vi "Log CAN messages.vi"(8 "error in":errorcluster, 9 "Period":i64, 10 "CAN Session In":T1, 11 "tdms file in":refnum<k34>) -> (0 "error out":errorcluster, 2 "CAN Session Out":T1, 3 "tdms file out":refnum<k34>)   [LabVIEW 2016]
uses:
  Program Files (x86)/National Instruments/LabVIEW 2016/examples/robotics/EPOS2 CANOpen Driver/Low Level VIs/Typedefs/CAN Refnum.ctl
  Program Files (x86)/National Instruments/LabVIEW 2016/examples/robotics/EPOS2 CANOpen Driver/Low Level VIs/Typedefs/CAN Session Pointer.ctl
  Program Files (x86)/National Instruments/LabVIEW 2016/examples/robotics/EPOS2 CANOpen Driver/Low Level VIs/Typedefs/CAN Communication References.ctl
  Program Files (x86)/National Instruments/LabVIEW 2016/examples/robotics/EPOS2 CANOpen Driver/Low Level VIs/Typedefs/kill process notifier array.ctl
  Program Files (x86)/National Instruments/LabVIEW 2016/examples/robotics/EPOS2 CANOpen Driver/Low Level VIs/Typedefs/Write Queue.ctl
  Program Files (x86)/National Instruments/LabVIEW 2016/examples/robotics/EPOS2 CANOpen Driver/Low Level VIs/Typedefs/FPGA CAN Frame Cluster.ctl
  <vilib>/Platform/TimedLoop/XDataNode/timing_clust.ctl
  <vilib>/Platform/TimedLoop/XDataNode/nitl_modes.ctl
  <vilib>/Platform/TimedLoop/XDataNode/wakeup.ctl
  <vilib>/Platform/TimedLoop/XDataNode/XDataNode.xnode
  <vilib>/Platform/TimedLoop/XDataNode/XDNodeRunTimeDep.lvlib
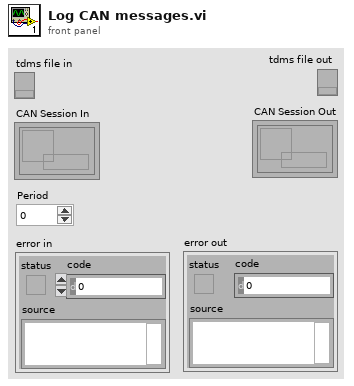
[diagram p1: front panel]
types:
  T1 = typedef "CAN Refnum.ctl" = refnum<k1>
  T2 = typedef "XDNodeRunTimeDep.lvlib/timing_clust.ctl" = cluster{"Expected End [f-1]":u64, "Actual End [f-1]":u64, "Finished Late? [f-1]":bool, "Expected End [i-1]":u64, "Actual End [i-1]":u64, "Finished Late? [i-1]":bool, "Expected Start [i]":u64, "Actual Start [i]":u64, "Expected Start [f]":u64, "Actual Start [f]":u64, "Source Name":string, "Structure Name":string, "Period":i64, "Deadline":i64, "Offset":i64, "Start":i64, "Priority":i32, "Timeout":i32, "Mode":T3, "Wakeup Reason":T4, "Error":errorcluster, "Source Type":string, "Secondary Source Type":string, "Global End Time":u64, "Global Start Time":u64, "Frame Duration":u64, "Iteration Duration":u64, "Assigned CPU":i32, "I/O Scan Engine Mode":u32}
  T3 = typedef "XDNodeRunTimeDep.lvlib/nitl_modes.ctl" = enum32{"No Change", "Process missed periods, maintain original phase", "Discard missed periods, maintain original phase", "Process missed periods, ignore original phase", "Discard missed periods, ignore original phase"}
  T4 = typedef "XDNodeRunTimeDep.lvlib/wakeup.ctl" = enum32{"Normal", "Aborted", "Asynchronous wakeup", "Timing source error", "Timed loop error", "Timeout"}
  T5 = typedef "FPGA CAN Frame Cluster.ctl" = cluster{"Timestamp":u64, "Identifier":u32, "Type":u8, "InfoA":u8, "InfoB":u8, "DataLength":u8, "Data":u8[]}
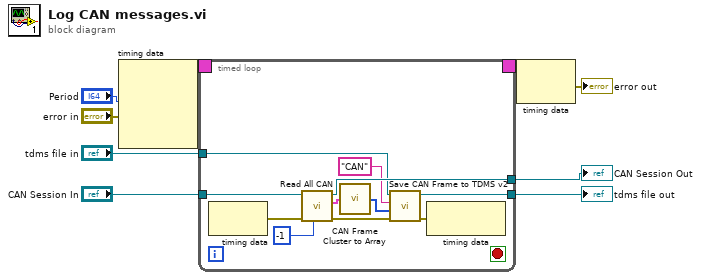
[diagram p0: block diagram]
diagram:
  n1 = node-c288("Period", "error in") -> (w5:T2)  [unwired: 2 in]
  n2 = timed-loop {
    timing: w5 -> [_]
    timing-out: [_] -> w4
    tunnel: "CAN Session In" -> [w19]
    tunnel: [w18] -> w8
    tunnel: "tdms file in" -> [w13]
    tunnel: [w12] -> w6
    stop <- _ stop-if-true
    n3 = node-c288() -> (w11:errorcluster)  [unwired: 1 in]
    n4 = call "Read All CAN.vi"("timeout in ms (-1)"=-1, "error in"=w11, "CAN Session In"=w19) -> ("error out"=w15:errorcluster, "CAN Frame Out"=w17:T5, "CAN Session Out"=w18:T1)  [unwired: 6 in]
    n5 = call "CAN Frame Cluster to Array.vi"("CAN Frame Cluster In"=w17) -> ("CAN Frame Array Out"=w16:u32[])
    n6 = call "Save CAN Frame to TDMS v2.vi"("tdms file in"=w13, "group name in"="CAN", "CAN Frame"=w16, "error in"=w15) -> ("tdms file out"=w12:refnum<k34>, "error out"=w10:errorcluster)  [unwired: 4 in, 1 out]
    n7 = node-c288(w10) -> ()  [unwired: 1 out]
  }
  "CAN Session Out" <- w8
  "tdms file out" <- w6
  n8 = node-c288(w4) -> (→"error out":errorcluster)
